vi "Sort downloaded image files.vi"() -> ()   [LabVIEW 2016]
panel:
  in  "Time Margin Sec":dbl=20.0
  out "Time difference in seconds":dbl[](array[numeric])
  out "Raw data filenames":path[](array[path])
  out "Raw Data Folder":path
  in  "Video folder camera downloads to":path=path "C:/Users/Paul Hayden/Pictures/Diplos flow vis/Camera_Downloads"
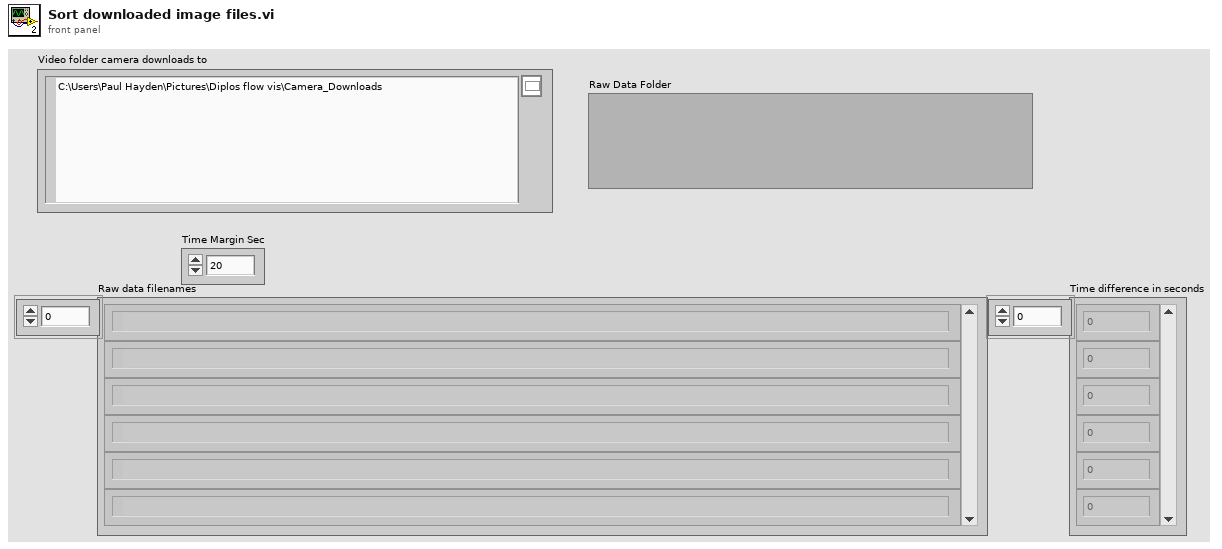
[diagram p1: front panel]
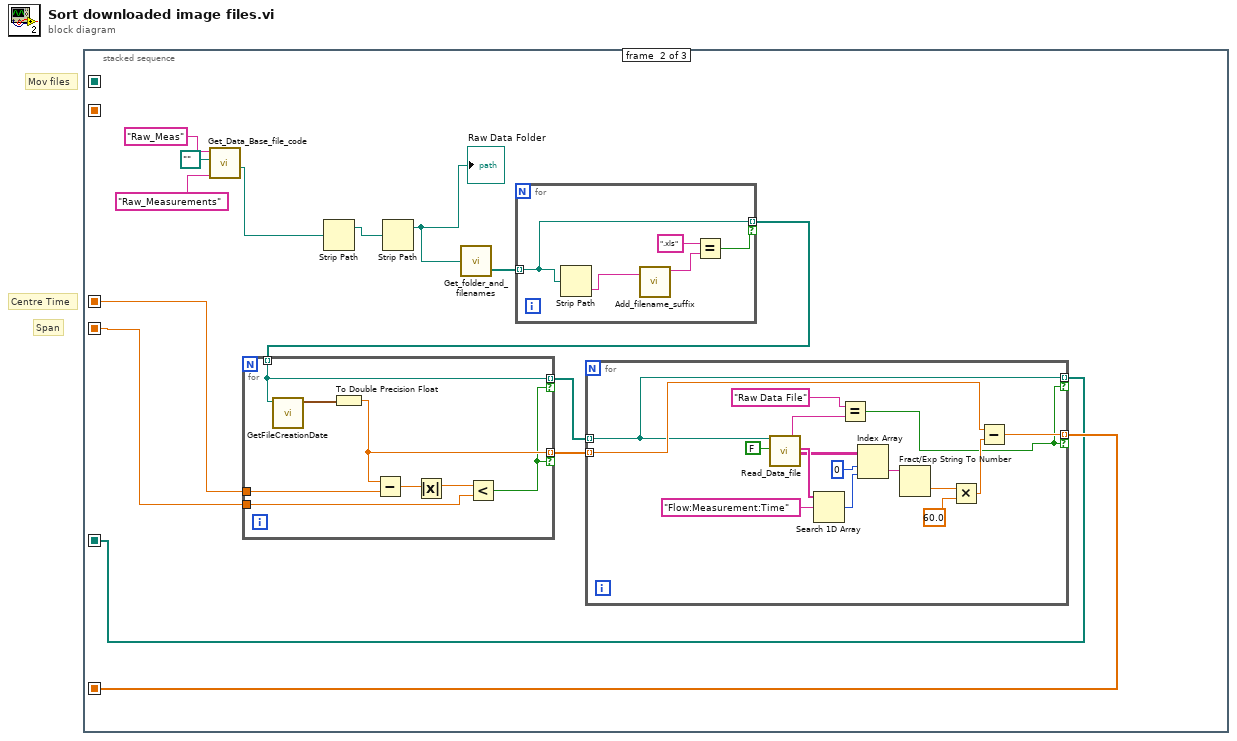
[diagram p0: block diagram]
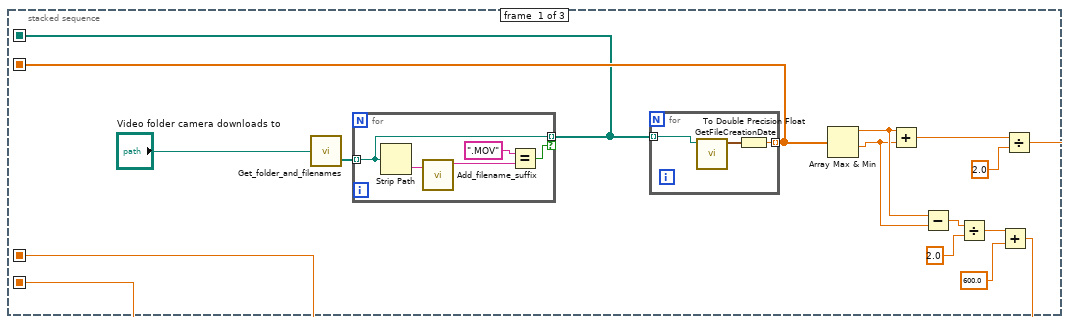
[diagram p2: hidden frame]
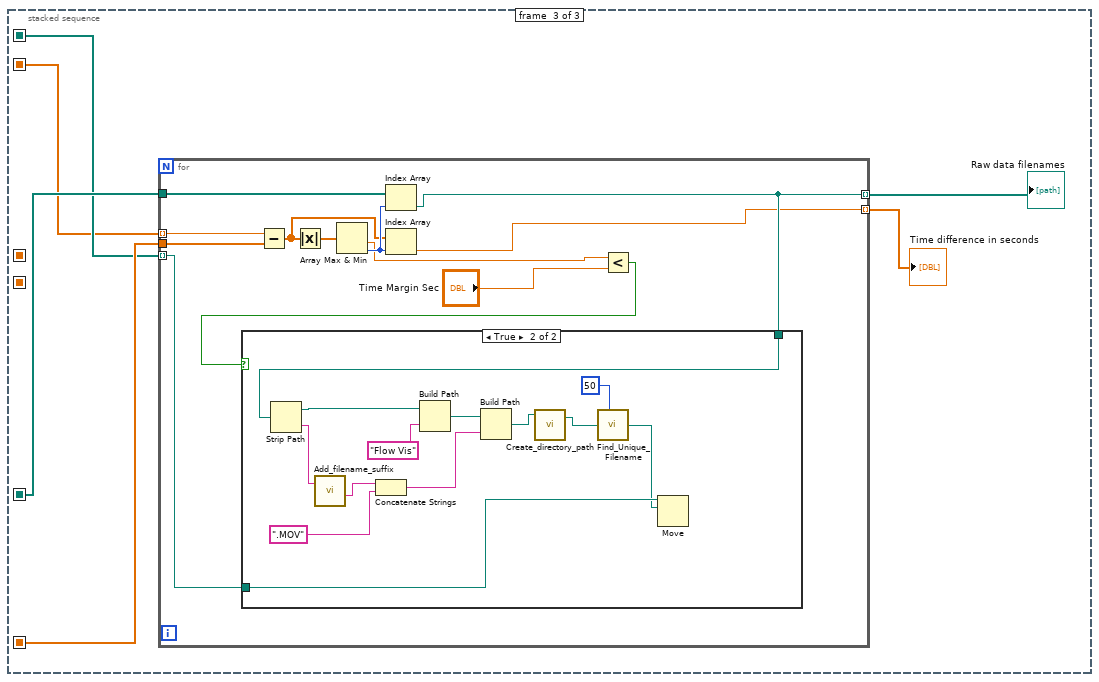
[diagram p3: hidden frame]
diagram:
  # "Mov files"
  # "Span"
  # "Centre Time"
  n1 = stacked-sequence {
    seq-local: [_ w24 _] -> [_ _ w71]
    seq-local: [_ w23 _] -> [_ _ w70]
    seq-local: [w4 _ _] -> [_ _ w66]
    seq-local: [w3 _ _] -> [_ w28 _]
    seq-local: [w2 _ _] -> [_ w27 _]
    seq-local: [w1 _ _] -> [_ _ w67]
    frame #0 {
      n2 = call "Get_folder_and_filenames.vi"("file path (dialog if empty)"="Video folder camera downloads to") -> ("Files"=w13:path[])  [unwired: 1 out]
      n3 = for {
        tunnel: w13 -> [w19] mode=indexing
        tunnel: [w19] -> w1 mode=indexing if=w18
        n4 = Strip Path(path=w19) -> (name=w22:string)  [unwired: 1 out]
        n5 = call "Add_filename_suffix.vi"("Filename"=w22) -> ("Original Suffix"=w21:string)  [unwired: 1 in, 3 out]
        n6 = Equal?(x=".MOV", y=w21) -> (x = y?=w18:bool)
      }
      n7 = for {
        tunnel: w1 -> [w17] mode=indexing
        tunnel: [w15] -> w4 mode=indexing
        n8 = call "GetFileCreationDate.vi"("File Path"=w17) -> ("File Created Date (UTC)"=w16:timestamp)  [unwired: 7 in, 1 out]
        n9 = To Double Precision Float(number=w16) -> (double precision float=w15:dbl)
      }
      n10 = Array Max & Min(array=w4) -> (max value=w10:dbl, min value=w9:dbl)  [unwired: 2 out]
      n11 = Add(x=w10, y=w9) -> (x+y=w12:dbl)
      n12 = Subtract(x=w10, y=w9) -> (x-y=w7:dbl)
      n13 = Divide(x=w7, y=2.0) -> (x/y=w6:dbl)
      n14 = Add(x=w6, y=600.0) -> (x+y=w2:dbl)
      n15 = Divide(x=w12, y=2.0) -> (x/y=w3:dbl)
    }
    frame #1 {
      n16 = call "Get_Data_Base_file_code.vi"("Data Type"="Raw_Measurements", "Results Filename"=path "", "Short_Name"="Raw_Meas") -> ("Raw Data File Name"=w32:path)  [unwired: 1 in, 3 out]
      n17 = Strip Path(path=w32) -> (stripped path=w33:path)  [unwired: 1 out]
      n18 = Strip Path(path=w33) -> (stripped path=w29:path)  [unwired: 1 out]
      "Raw Data Folder" <- w29
      n19 = call "Get_folder_and_filenames.vi"("file path (dialog if empty)"=w29) -> ("Files"=w31:path[])  [unwired: 1 out]
      n20 = for {
        tunnel: w31 -> [w62] mode=indexing
        tunnel: [w62] -> w30 mode=indexing if=w61
        n21 = Strip Path(path=w62) -> (name=w65:string)  [unwired: 1 out]
        n22 = call "Add_filename_suffix.vi"("Filename"=w65) -> ("Original Suffix"=w64:string)  [unwired: 1 in, 3 out]
        n23 = Equal?(x=".xls", y=w64) -> (x = y?=w61:bool)
      }
      n24 = for {
        tunnel: w30 -> [w55] mode=indexing
        tunnel: w28 -> [w59]
        tunnel: w27 -> [w56]
        tunnel: [w55] -> w26 mode=indexing if=w53
        tunnel: [w54] -> w25 mode=indexing if=w53
        n25 = call "GetFileCreationDate.vi"("File Path"=w55) -> ("File Created Date (UTC)"=w60:timestamp)  [unwired: 7 in, 1 out]
        n26 = To Double Precision Float(number=w60) -> (double precision float=w54:dbl)
        n27 = Subtract(x=w54, y=w59) -> (x-y=w58:dbl)
        n28 = Absolute Value(x=w58) -> (abs(x)=w57:dbl)
        n29 = Less?(x=w57, y=w56) -> (x < y?=w53:bool)
      }
      n30 = for {
        tunnel: w26 -> [w39] mode=indexing
        tunnel: w25 -> [w42] mode=indexing
        tunnel: [w40] -> w24 mode=indexing if=w38
        tunnel: [w39] -> w23 mode=indexing if=w38
        n31 = call "Read_Data_file.vi"("Results file"=w39, "Delete First Rows?"=FALSE) -> ("Filetype"=w46:string, "Ch names Out"=w52:string[], "Channel Values Out"=w50:string[][])  [unwired: 7 in, 8 out]
        n32 = Search 1D Array(1D array=w52, element="Flow:Measurement:Time") -> (index of element=w48:i32)  [unwired: 1 in]
        n33 = Equal?(x="Raw Data File", y=w46) -> (x = y?=w38:bool)
        n34 = Index Array(array=w50, index (row)=0, index (col)=w48) -> (element=w47:string)
        n35 = Fract/Exp String To Number(string=w47) -> (number=w43:dbl)  [unwired: 3 in, 1 out]
        n36 = Multiply(x=w43, y=60.0) -> (x*y=w41:dbl)
        n37 = Subtract(x=w42, y=w41) -> (x-y=w40:dbl)
      }
    }
    frame #2 {
      n38 = for {
        tunnel: w67 -> [w77] mode=indexing
        tunnel: w71 -> [w83]
        tunnel: w70 -> [w81]
        tunnel: [w78] -> w69 mode=indexing
        tunnel: [w72] -> w68 mode=indexing
        tunnel: w66 -> [w76] mode=indexing
        n39 = Subtract(x=w76, y=w83) -> (x-y=w79:dbl[])
        n40 = Absolute Value(x=w79) -> (abs(x)=w82:dbl[])
        n41 = Array Max & Min(array=w82) -> (min value=w75:dbl, min index (indices)=w80:i32)  [unwired: 2 out]
        n42 = Index Array(array=w81, index=w80) -> (element=w78:path)
        n43 = Index Array(array=w79, index=w80) -> (element=w72:dbl)
        n44 = Less?(x=w75, y="Time Margin Sec") -> (x < y?=w73:bool)
        n45 = case shown="True" w73 {
          tunnel: w78 -> [_ w96]
          tunnel: w77 -> [_ w91]
          frame False {
          }
          frame True {
            n46 = Strip Path(path=w96) -> (stripped path=w84:path, name=w94:string)
            n47 = call "Add_filename_suffix.vi"("Filename"=w94) -> ("Base name"=w87:string)  [unwired: 1 in, 3 out]
            n48 = Concatenate Strings(w87, ".MOV" ("x")) -> (w85:string)
            n49 = Build Path(base path=w84, name or relative path="Flow Vis") -> (appended path=w93:path)
            n50 = Build Path(base path=w93, name or relative path=w85) -> (appended path=w89:path)
            n51 = call "Create_directory_path.vi"("Path name"=w89) -> ("Path name Out"=w88:path)  [unwired: 2 in, 1 out]
            n52 = call "Find_Unique_Filename.vi"("Path In"=w88, "Max Length (31)"=50) -> ("Unique Path Out"=w90:path)  [unwired: 1 in]
            n53 = Move(source path=w91, 10:w90) -> ()  [unwired: 3 in, 3 out]
          }
        }
      }
      "Raw data filenames" <- w69
      "Time difference in seconds" <- w68
    }
  }
